vi "Open File to Log.vi"(8 "error in (no error)":errorcluster, 11 "File Path":path) -> (0 "error out":errorcluster, 2 "pcap dumper_reference":u64, 3 "pcap reference":u64)   [LabVIEW 2025, in "Automotive Ethernet Bus Monitor UI.lvlib" / "lvwpcap.lvlib"]
uses:
  lvwpcap.lvlib
  lvwpcap.dll
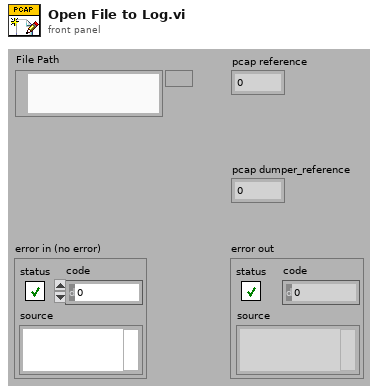
[diagram p1: front panel]
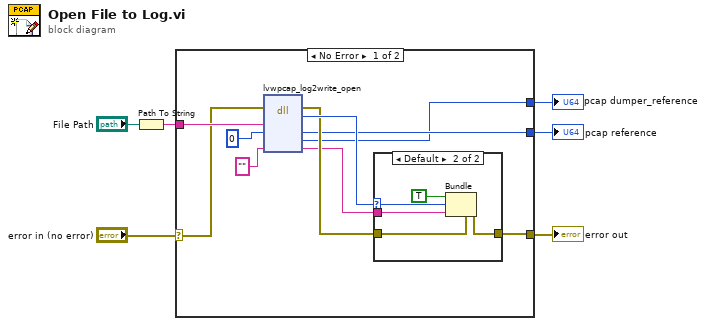
[diagram p0: block diagram]
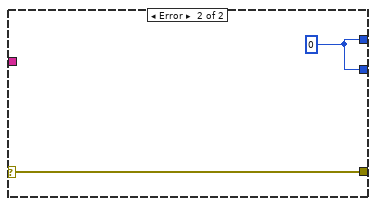
[diagram p3: hidden frame]
diagram:
  n1 = Path To String(path="File Path") -> (string=w4:string)
  n2 = case shown="No Error" "error in (no error)" {
    selector: "error in (no error)" -> [w14 w24]
    tunnel: [w12 w24] -> w6
    tunnel: [w11 w23] -> w2
    tunnel: w4 -> [w16 _]
    tunnel: [w7 w23] -> w1
    frame No Error {
      n3 = dll-call lib="lvwpcap.*" fn="lvwpcap_log2write_open"(error in=w14, "file_path"=w16, "pcap"=u64 0, "error_string"="") -> (error out=w13:errorcluster, "return type"=w15:u64, "pcap"=w11:u64, "pcap_dumper"=w7:u64, "error_string"=w10:string)  [unwired: 4 in, 1 out]
      n4 = case shown="Default" w15 {
        selector: w15 -> [_ w21]
        tunnel: w10 -> [_ w20]
        tunnel: w13 -> [w17 w22]
        tunnel: [w17 w18] -> w12
        frame 0 {
        }
        frame Default {
          n5 = Bundle(cluster=w22, "status"=TRUE, "code"=w21, "source"=w20) -> (w18:errorcluster)
        }
      }
    }
    frame Error {
      w23 = u64 0 ("pcap")
    }
  }
  "error out" <- w6
  "pcap reference" <- w2
  "pcap dumper_reference" <- w1
